vi "scan sys config device information.vi"(8 "error in":errorcluster, 11 "system session in":refnum<k21>) -> (0 "error out":errorcluster, 2 "controller information":T1 {"product ID" format="%.0x"; "primary network adapter"."IP address request mode" items=["Static"=1, "DHCP/Link Local"=2, "Link-Local Only"=4, "DHCP Only"=8]; "primary network adapter"."adapter type" items=["Ethernet"=1, "WLAN"=2]; "primary network adapter"."adapter mode" items=["Disabled"=1, "TCP/IP Ethernet"=2, "Deterministic"=4, "EtherCAT"=8, "TCP/IP WLAN Connect"=32, "TCP/IP WLAN Create"=64]; "secondary network adapters"."IP address request mode" items=["Static"=1, "DHCP/Link Local"=2, "Link-Local Only"=4, "DHCP Only"=8]; "secondary network adapters"."adapter type" items=["Disabled"=1, "TCP/IP Ethernet"=2, "Deterministic"=4, "EtherCAT"=8, "TCP/IP WLAN Connect"=32, "TCP/IP WLAN Create"=64]; "secondary network adapters"."adapter mode" items=["Disabled"=1, "TCP/IP Ethernet"=2, "Deterministic"=4, "EtherCAT"=8, "TCP/IP WLAN Connect"=32, "TCP/IP WLAN Create"=64]}, 3 "system session out":refnum<k21>)   [LabVIEW 2014, in "SMI.lvlib" / "Controller.lvclass"]
uses:
  Controller.lvclass
  controller information.ctl
  device information.ctl
  network adapter settings.ctl
  <vilib>/nisyscfg/Find Hardware.vi
  <vilib>/nisyscfg/Close (Resources).vi
  <vilib>/nisyscfg/Close (Filter).vi
  <resource>/objmgr/niflexriosae.rc
  <vilib>/nisyscfg/nisyscfg.lvlib
  <resource>/objmgr/nisysapi.rc
  SMI.lvlib
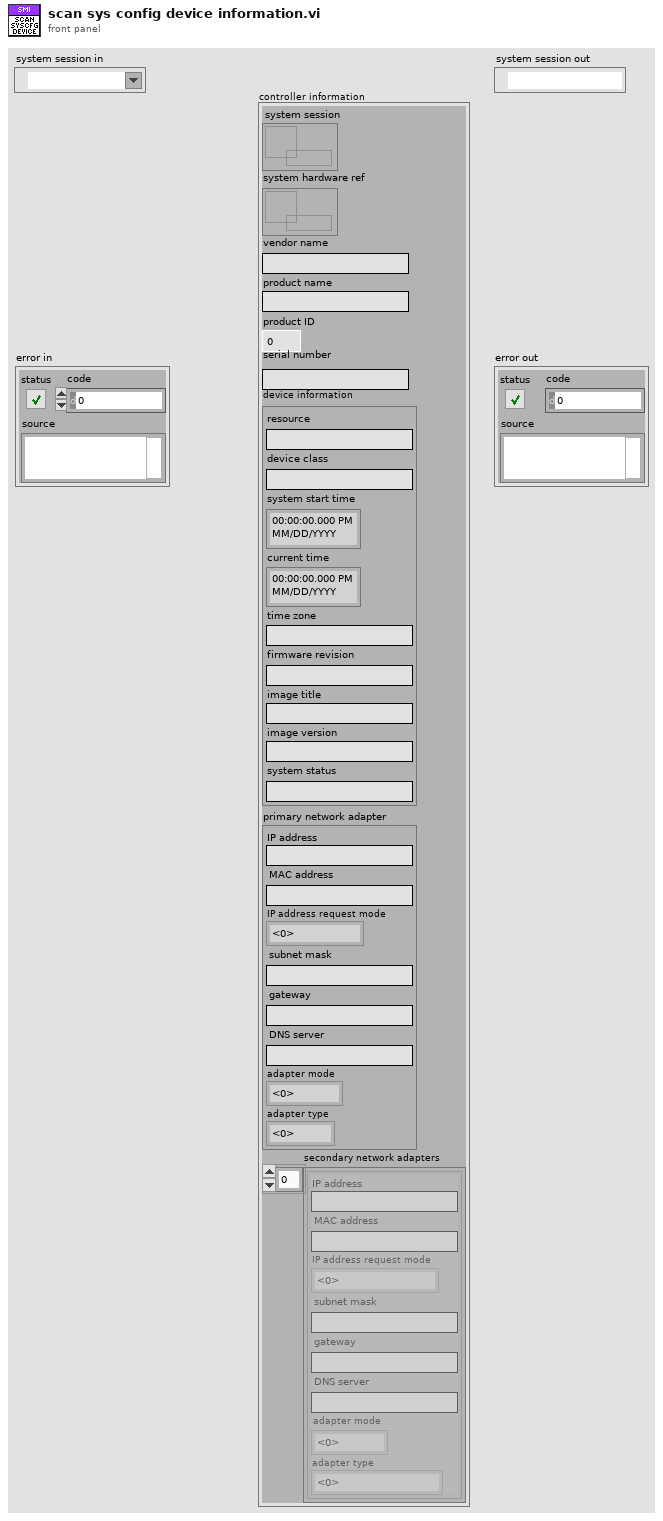
[diagram p1: front panel]
types:
  T1 = typedef "SMI.lvlib/Controller.lvclass/controller information.ctl" = cluster{"system session":refnum<data-value>, "system hardware ref":refnum<data-value>, "vendor name":string, "product name":string, "product ID":u16, "serial number":string, "device information":T2, "primary network adapter":T3, "secondary network adapters":T3[]}
  T2 = typedef "SMI.lvlib/Controller.lvclass/device information.ctl" = cluster{"resource":string, "device class":string, "system start time":timestamp, "current time":timestamp, "time zone":string, "firmware revision":string, "image title":string, "image version":string, "system status":string}
  T3 = typedef "SMI.lvlib/Controller.lvclass/network adapter settings.ctl" = cluster{"IP address":string, "MAC address":string, "IP address request mode":u32, "subnet mask":string, "gateway":string, "DNS server":string, "adapter mode":u32, "adapter type":u32}
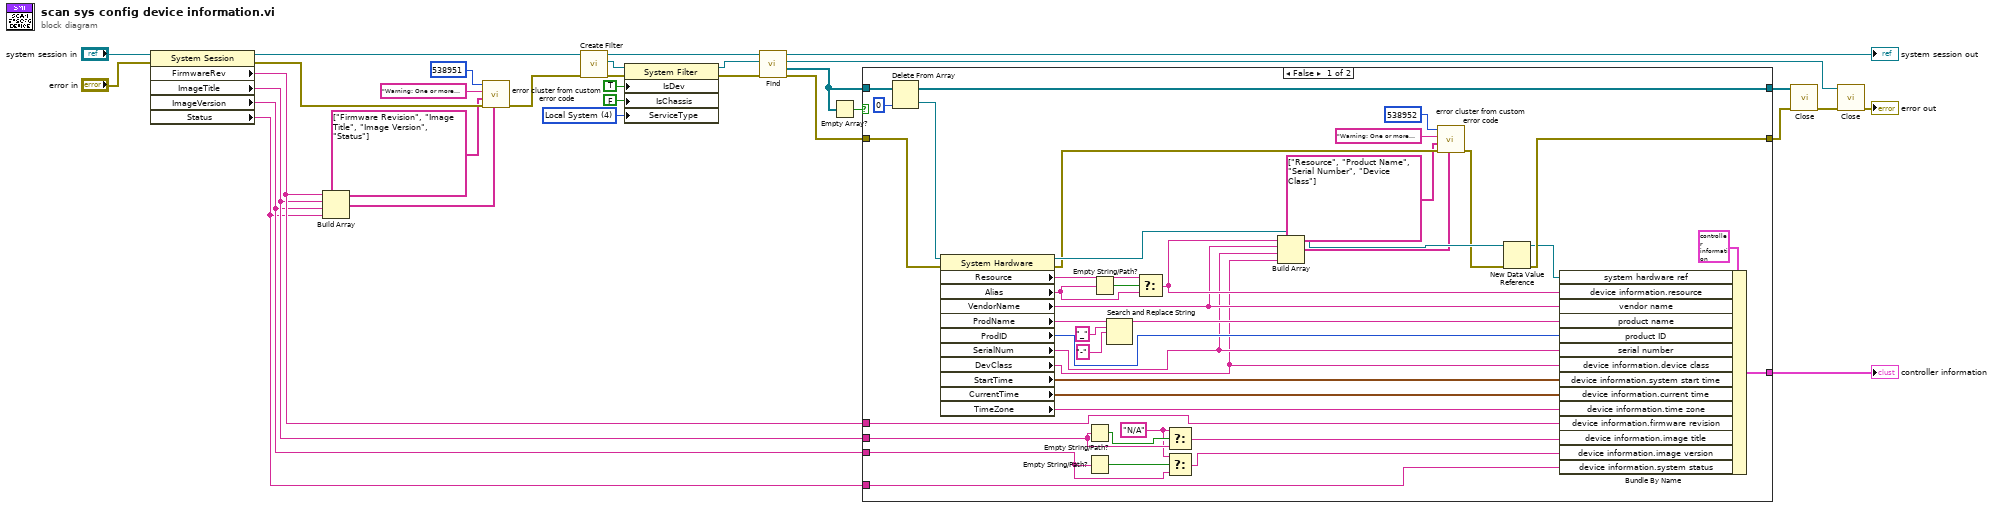
[diagram p0: block diagram]
diagram:
  w10 = u32 4 items=["NI Network Resource", "NI Real-Time", "NI System Configuration", "NI Web Interface", "Local System", "Local Network Adapter", "Local Time Keeper", "Local Time Reference", "LXI Instrument", "Local FPGA"] ("Service Type")
  n1 = property class="System Session"(reference="system session in", error in="error in") -> (reference out=w27:refnum<k21>, error out=w20:errorcluster, "FirmwareRev"=w8:string, "ImageTitle"=w7:string, "ImageVersion"=w6:string, "Status"=w5:string)
  n2 = Build Array(w8, w7, w6, w5) -> (w2:string[])
  n3 = call "error cluster from custom error code.vi"("string values"=w2, "error in"=w20, "keys"=string[] ["Firmware Revision", "Image Title", "Image Version", "Status"], "error message"="Warning: One or more System Session properties are not available for the target.", "custom error code (0)"=538951 ("error code (0)")) -> ("error out"=w26:errorcluster)  [unwired: 6 in]
  n4 = call <vilib>:"Create Filter.vi"("error in (no error)"=w26, "Session in"=w27) -> ("error out"=w11:errorcluster, "Filter out"=w12:refnum<k20>, "Session out"=w28:refnum<k21>)  [unwired: 7 in]
  n5 = property class="System Filter"(reference=w12, error in=w11, "IsDev"=TRUE ("Is Device"), "IsChassis"=FALSE ("Is Chassis"), "ServiceType"=w10) -> (reference out=w29:refnum<k20>, error out=w25:errorcluster)
  n6 = call-poly <vilib>:"Find.vi"("error in (no error)"=w25, "Filter in"=w29, "Session in"=w28) -> ("error out"=w24:errorcluster, "Resources out"=w18:refnum<k20>[], "Filter out"=w23:refnum<k20>, "Session out"=→"system session out":refnum<k21>)  [unwired: 5 in]
  n7 = Empty Array?(array=w18) -> (empty?=w17:bool)
  n8 = case shown="False" w17 {
    tunnel: w24 -> [w71 w72]
    tunnel: w8 -> [w70 _]
    tunnel: [w43 w72] -> w14
    tunnel: w7 -> [w69 _]
    tunnel: w5 -> [w68 _]
    tunnel: w6 -> [w67 _]
    tunnel: [w66 _] -> w19
    tunnel: w18 -> [w47 w73]
    tunnel: [w45 w73] -> w16
    frame False {
      w51 = "N/A"
      n9 = Delete From Array(array=w47, index=0) -> (deleted portion=w46:refnum<k20>, array with subset deleted=w45:refnum<k20>[])  [unwired: 1 in]
      n10 = property class="System Hardware"(reference=w46, error in=w71) -> (reference out=w44:refnum<k20>, error out=w36:errorcluster, "Resource"=w62:string, "Alias"=w61:string, "VendorName"=w39:string, "ProdName"=w58:string, "ProdID"=w56:u32, "SerialNum"=w38:string, "DevClass"=w37:string, "StartTime"=w59:timestamp, "CurrentTime"=w63:timestamp, "TimeZone"=w64:string)
      n11 = Empty String/Path?(string/path=w69) -> (empty?=w52:bool)
      n12 = Empty String/Path?(string/path=w67) -> (empty?=w53:bool)
      n13 = Empty String/Path?(string/path=w61) -> (empty?=w60:bool)
      n14 = Search and Replace String(input string=w58, search string="_", replace string="-" ("replace string (\"\")")) -> (result string=w57:string)  [unwired: 5 in, 3 out]
      n15 = Select(t=w62, s=w60, f=w61) -> (s? t:f=w40:string)
      n16 = Select(t=w51, s=w52, f=w69) -> (s? t:f=w49:string)
      n17 = Select(t=w51, s=w53, f=w67) -> (s? t:f=w50:string)
      n18 = Build Array(w40, w39, w38, w37) -> (w34:string[])
      n19 = call "error cluster from custom error code.vi"("string values"=w34, "error in"=w36, "keys"=string[] ["Resource", "Product Name", "Serial Number", "Device Class"], "error message"="Warning: One or more System Hardware properties are not available for the target.", "custom error code (0)"=538952 ("error code (0)")) -> ("error out"=w42:errorcluster)  [unwired: 6 in]
      n20 = New Data Value Reference(data value=w44, error in=w42) -> (data value reference=w41:refnum<data-value>, error out=w43:errorcluster)
      n21 = Bundle By Name(cluster=T1 {"system session"=refnum, "system hardware ref"=refnum, "vendor name"="", "product name"="", "product ID"=0, "serial number"="", "device information"={"resource"="", "device class"="", "system start time"=timestamp(0 s since 1904-01-01), "current time"=timestamp(0 s since 1904-01-01), "time zone"="", "firmware revision"="", "image title"="", "image version"="", "system status"=""}, "primary network adapter"={"IP address"="", "MAC address"="", "IP address request mode"=1, "subnet mask"="", "gateway"="", "DNS server"="", "adapter mode"=1, "adapter type"=1}, "secondary network adapters"=[]} ("Network Device"), "system hardware ref"=w41, "device information.resource"=w40, "vendor name"=w39, "product name"=w57, "product ID"=w56, "serial number"=w38, "device information.device class"=w37, "device information.system start time"=w59, "device information.current time"=w63, "device information.time zone"=w64, "device information.firmware revision"=w70, "device information.image title"=w49, "device information.image version"=w50, "device information.system status"=w68) -> (w66:T1)
    }
    frame True {
    }
  }
  "controller information" <- w19
  n22 = call-poly <vilib>:"Close.vi"("error in (no error)"=w14, "Resources in"=w16) -> ("error out"=w15:errorcluster)  [unwired: 9 in]
  n23 = call-poly <vilib>:"Close.vi"("error in (no error)"=w15, "Filter in"=w23) -> ("error out"=→"error out":errorcluster)  [unwired: 9 in]
